vi "DeleteEmptyStreamFolders.vi"(8 "error in (no error)":errorcluster, 9 "data group":string, 10 "stream Id":string) -> (0 "error out":errorcluster)   [LabVIEW 2017, in "FileManager.lvlib"]
uses:
  <vilib>/addons/InsightCM/Devices/Shared/Common/FileManager/FileManager.lvlib
  <vilib>/addons/InsightCM/Utilities/GlobalConfiguration/GlobalConfiguration.lvlib
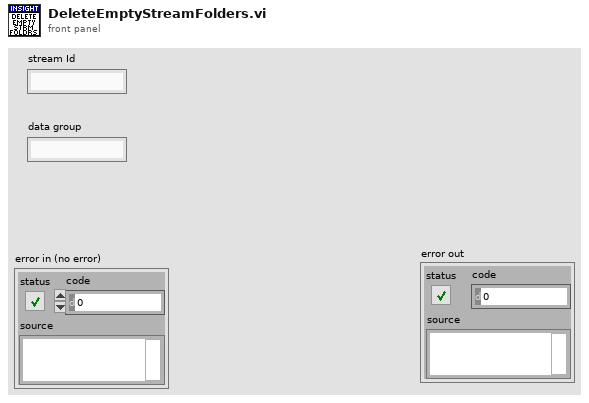
[diagram p1: front panel]
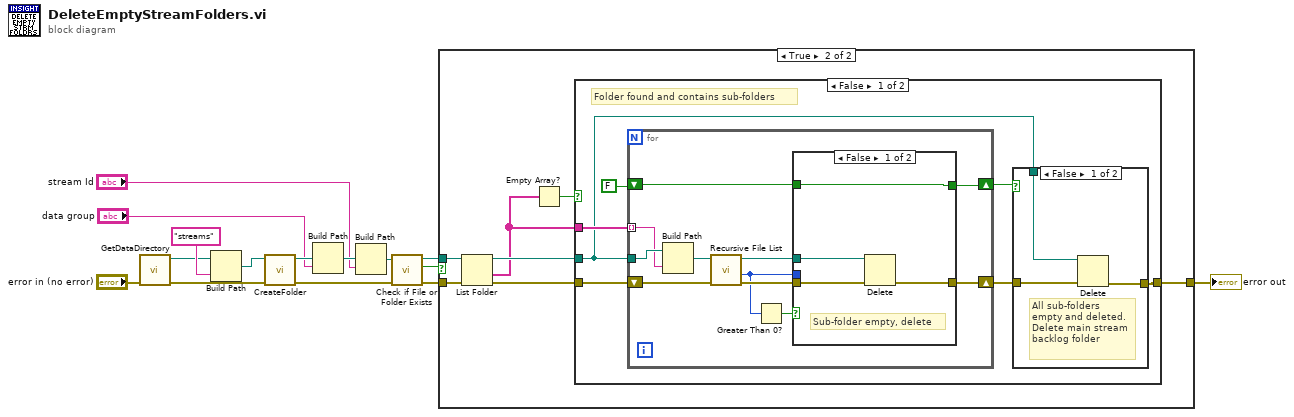
[diagram p0: block diagram]
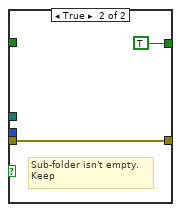
[diagram p4: hidden frame]
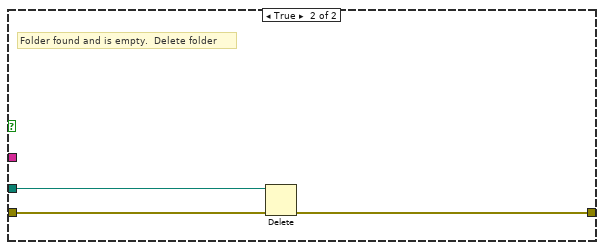
[diagram p5: hidden frame]
diagram:
  n1 = call <vilib>:"GetDataDirectory.vi"("error in (no error)"="error in (no error)") -> ("error out"=w11:errorcluster, "data directory"=w10:path)  [unwired: 9 in]
  n2 = Build Path(base path=w10, name or relative path="streams") -> (appended path=w13:path)
  n3 = call <vilib>:"CreateFolder.vi"("error in (no error)"=w11, "folder"=w13) -> ("error out"=w8:errorcluster, "folder out"=w9:path)  [unwired: 8 in]
  n4 = Build Path(base path=w9, name or relative path="data group") -> (appended path=w4:path)
  n5 = Build Path(base path=w4, name or relative path="stream Id") -> (appended path=w3:path)
  n6 = call <vilib>:"Check if File or Folder Exists.vi"("error in (no error)"=w8, "path"=w3) -> ("error out"=w7:errorcluster, "file or folder exists?"=w5:bool, "dup path"=w6:path)  [unwired: 7 in]
  n7 = case shown="True" w5 {
    tunnel: [w16 w23] -> w15
    tunnel: w7 -> [w16 w18]
    tunnel: w6 -> [_ w17]
    frame False {
      # "No folder with stream Id found"
    }
    frame True {
      n8 = List Folder(path=w17, error in=w18) -> (path out=w21:path, folder names=w20:string[], error out=w22:errorcluster)  [unwired: 1 in, 2 out]
      n9 = Empty Array?(array=w20) -> (empty?=w19:bool)
      n10 = case shown="False" w19 {
        tunnel: [w27 w53] -> w23
        tunnel: w22 -> [w30 w54]
        tunnel: w21 -> [w26 w52]
        tunnel: w20 -> [w29 _]
        frame False {
          # "Folder found and contains sub-folders"
          n11 = for {
            shift-right: [w45] -> w28
            shift-left: w30 -> [w44]
            tunnel: w29 -> [w42] mode=indexing
            tunnel: w26 -> [w43]
            shift-right: [w35] -> w24
            shift-left: FALSE -> [w36]
            n12 = Build Path(base path=w43, name or relative path=w42) -> (appended path=w41:path)
            n13 = call <vilib>:"Recursive File List.vi"("error in (no error)"=w44, "Folder Path"=w41) -> ("error out"=w40:errorcluster, "Number of Files"=w39:i32, "dup Folder Path"=w37:path)  [unwired: 5 in, 2 out]
            n14 = Greater Than 0?(x=w39) -> (x > 0?=w38:bool)
            n15 = case shown="False" w38 {
              tunnel: [w48 w51] -> w45
              tunnel: w40 -> [w49 w51]
              tunnel: w39 -> [_ _]
              tunnel: w37 -> [w47 _]
              tunnel: w36 -> [w46 _]
              tunnel: [w46 TRUE] -> w35
              frame False {
                # "Sub-folder empty, delete"
                n16 = Delete(path (use dialog)=w47, error in=w49) -> (error out=w48:errorcluster)  [unwired: 3 in, 2 out]
              }
              frame True {
                # "Sub-folder isn't empty.\nKeep"
              }
            }
          }
          n17 = case shown="False" w24 {
            tunnel: w28 -> [w33 w34]
            tunnel: [w32 w34] -> w27
            tunnel: w26 -> [w31 _]
            frame False {
              # "All sub-folders\nempty and deleted.\nDelete main stream\nbacklog folder"
              n18 = Delete(path (use dialog)=w31, error in=w33) -> (error out=w32:errorcluster)  [unwired: 3 in, 2 out]
            }
            frame True {
            }
          }
        }
        frame True {
          # "Folder found and is empty.  Delete folder"
          n19 = Delete(path (use dialog)=w52, error in=w54) -> (error out=w53:errorcluster)  [unwired: 3 in, 2 out]
        }
      }
    }
  }
  "error out" <- w15
